vi "Read All CAN.vi"(6 "timeout in ms (-1)":i32, 8 "error in":errorcluster, 11 "CAN Session In":T2) -> (0 "error out":errorcluster, 2 "CAN Frame Out":T1 {"Data" format="%.0x"; "DataLength" format="%.0x"; "InfoB" format="%.0x"; "InfoA" format="%.0x"; "Type" format="%.0x"; "Identifier" format="%.0x"; "Timestamp" format="%.0x"}, 3 "CAN Session Out":T2)   [LabVIEW 2016]
doc: "The VI read a CAN packet (frame) from the CAN bus."
uses:
  Program Files (x86)/National Instruments/LabVIEW 2016/examples/robotics/EPOS2 CANOpen Driver/Low Level VIs/Typedefs/CAN Refnum.ctl
  Program Files (x86)/National Instruments/LabVIEW 2016/examples/robotics/EPOS2 CANOpen Driver/Low Level VIs/Typedefs/CAN Session Pointer.ctl
  Program Files (x86)/National Instruments/LabVIEW 2016/examples/robotics/EPOS2 CANOpen Driver/Low Level VIs/Typedefs/CAN Communication References.ctl
  Program Files (x86)/National Instruments/LabVIEW 2016/examples/robotics/EPOS2 CANOpen Driver/Low Level VIs/Typedefs/kill process notifier array.ctl
  Program Files (x86)/National Instruments/LabVIEW 2016/examples/robotics/EPOS2 CANOpen Driver/Low Level VIs/Typedefs/Write Queue.ctl
  Program Files (x86)/National Instruments/LabVIEW 2016/examples/robotics/EPOS2 CANOpen Driver/Low Level VIs/Typedefs/FPGA CAN Frame Cluster.ctl
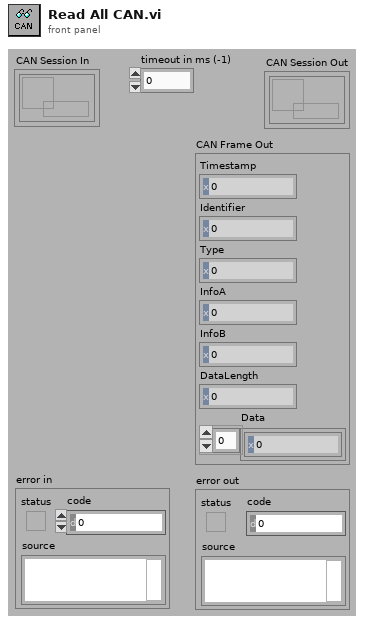
[diagram p1: front panel]
types:
  T1 = typedef "FPGA CAN Frame Cluster.ctl" = cluster{"Timestamp":u64, "Identifier":u32, "Type":u8, "InfoA":u8, "InfoB":u8, "DataLength":u8, "Data":u8[]}
  T2 = typedef "CAN Refnum.ctl" = refnum<k1>
  T3 = typedef "Write Queue.ctl" = refnum<queue>
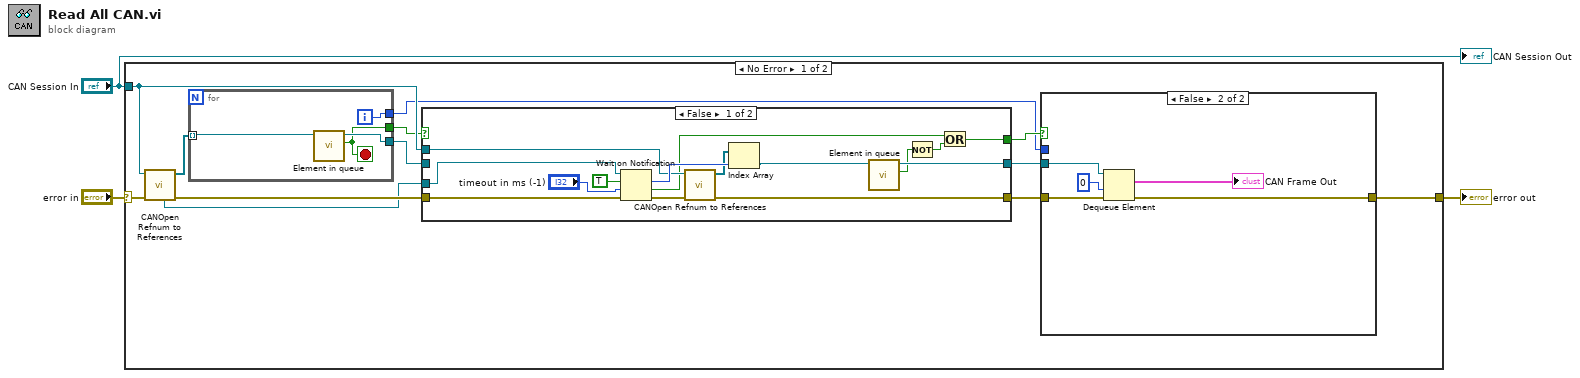
[diagram p0: block diagram]
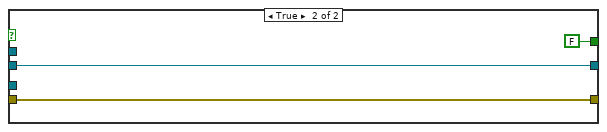
[diagram p2: hidden frame]
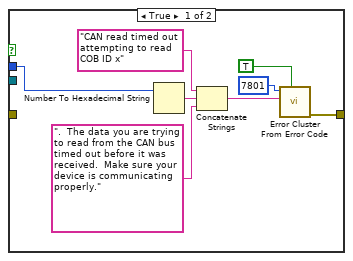
[diagram p3: hidden frame]
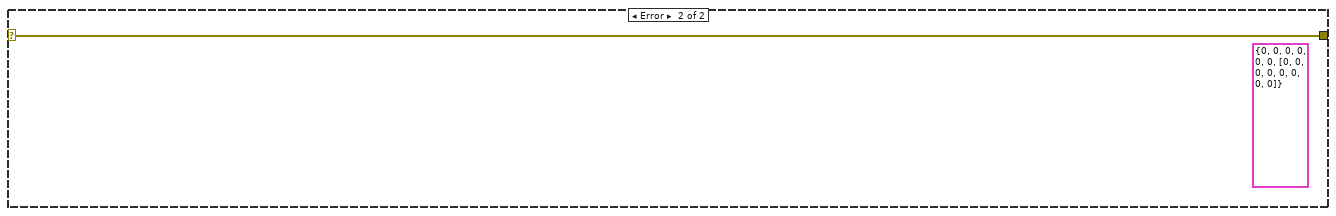
[diagram p4: hidden frame]
diagram:
  n1 = case shown="No Error" "error in" {
    selector: "error in" -> [w14 w51]
    tunnel: [w11 w51] -> w3
    tunnel: "CAN Session In" -> [w15 _]
    frame No Error {
      n2 = call "CANOpen Refnum to References.vi"("error in (no error)"=w14, "CAN Session In"=w15) -> ("error out"=w10:errorcluster, "Read Queue Array"=w6:T3[], "New Frame Notifier"=w9:refnum<notifier>)  [unwired: 7 out]
      n3 = for {
        tunnel: w6 -> [w34] mode=indexing
        tunnel: [w37] -> w7
        tunnel: [w36] -> w8
        tunnel: [w35] -> w4
        i -> [w35]
        stop <- w36 stop-if-true
        n4 = call "Element in queue.vi"("queue"=w34) -> ("Ready to read"=w36:bool, "queue out"=w37:T3)  [unwired: 9 in]
      }
      n5 = case shown="False" w8 {
        tunnel: w10 -> [w30 w32]
        tunnel: [w23 w32] -> w13
        tunnel: w9 -> [w29 _]
        tunnel: [w21 w33] -> w12
        tunnel: w7 -> [_ w33]
        tunnel: w15 -> [w26 _]
        tunnel: [w17 FALSE ("timed out?")] -> w5
        frame False {
          n6 = Wait on Notification(notifier=w29, ignore previous (F)=TRUE, timeout in ms (-1)="timeout in ms (-1)", error in (no error)=w30) -> (notification=w27:i32, timed out?=w18:bool, error out=w25:errorcluster)  [unwired: 1 out]
          n7 = call "CANOpen Refnum to References.vi"("error in (no error)"=w25, "CAN Session In"=w26) -> ("error out"=w23:errorcluster, "Read Queue Array"=w24:T3[])  [unwired: 8 out]
          n8 = Index Array(array=w24, index=w27) -> (element=w16:T3)
          n9 = call "Element in queue.vi"("queue"=w16) -> ("Ready to read"=w19:bool, "queue out"=w21:T3)  [unwired: 9 in]
          n10 = Not(x=w19) -> (.not. x?=w20:bool)
          n11 = Or(x=w18, y=w20) -> (x .or. y?=w17:bool)
        }
        frame True {
        }
      }
      n12 = case shown="False" w5 {
        tunnel: [w41 w48] -> w11
        tunnel: w13 -> [_ w47]
        tunnel: w12 -> [_ w49]
        tunnel: w4 -> [w38 _]
        frame True {
          n13 = Number To Hexadecimal String(2:w38) -> (0:w39:string)  [unwired: 1 in]
          n14 = Concatenate Strings("CAN read timed out attempting to read COB ID x", w39, ".  The data you are trying to read from the CAN bus timed out before it was received.  Make sure your device is communicating properly.") -> (w43:string)
          n15 = call <vilib>:"Error Cluster From Error Code.vi"("show call chain? (False)"=TRUE, "error message (\"\")"=w43, "error code (0)"=7801) -> ("error out"=w41:errorcluster)  [unwired: 1 in, 5 out]
        }
        frame False {
          n16 = Dequeue Element(queue=w49, timeout in ms (-1)=0, error in (no error)=w47) -> (element=→"CAN Frame Out":T1, error out=w48:errorcluster)  [unwired: 2 out]
        }
      }
    }
    frame Error {
      (unwired) T1 {"Timestamp"=0, "Identifier"=0, "Type"=0, "InfoA"=0, "InfoB"=0, "DataLength"=0, "Data"=[0, 0, 0, 0, 0, 0, 0, 0]} ("CAN Frame")
    }
  }
  "error out" <- w3
  "CAN Session Out" <- "CAN Session In"
